vi "Confirm Device UI.vi"(11 "Device":refnum<class "Device.lvclass">) -> (3 "Confirmed":bool)   [LabVIEW 2020, in "PicoG-App.lvlib" / "picoG.lvclass"]
uses:
  picoG.lvclass
  Device/Device.lvclass
panel:
  out "Picture":picture
  in  "Cancel Button":bool
  in  "OK Button":bool
  out "Version":string
  out "Name":string
  out "Id / Serial":string
  out "Board":string
  out "Platform":string
  # "Confirm device selection to continue adding the device to the registry.\n\nIf desired, the alias can be changed once the device is added."
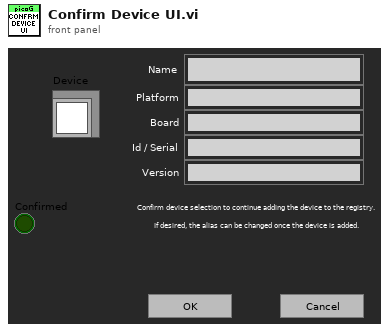
[diagram p1: front panel]
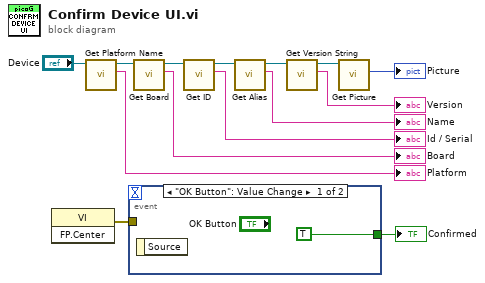
[diagram p0: block diagram]
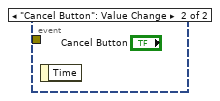
[diagram p2: hidden frame]
diagram:
  n1 = invoke class="VI" method="FP.Center"() -> (error out=w3:errorcluster)  [unwired: 3 in, 2 out]
  n2 = call "Get Platform Name.vi"("Device in"="Device") -> ("Platform"=→"Platform":string, "Device out"=w13:refnum<class "Device.lvclass">)  [unwired: 8 in, 1 out]
  n3 = event shown="[0] \"OK Button\": Value Change" {
    selector: _ -> [_ _]
    dyn-events: _ -> [_ _]
    timeout: _ -> [_ _]
    tunnel: [TRUE _] -> w4
    tunnel: w3 -> [_ _]
    event "OK Button": Value Change {
      n4 = event-data() -> ()  [unwired: 1 in, 1 out]
    }
    event "Cancel Button": Value Change {
      n5 = event-data() -> ()  [unwired: 1 in, 1 out]
    }
  }
  "Confirmed" <- w4
  n6 = call "Get Board.vi"("Device in"=w13) -> ("Board"=→"Board":string, "Device out"=w12:refnum<class "Device.lvclass">)  [unwired: 8 in, 1 out]
  n7 = call "Get ID.vi"("Device in"=w12) -> ("Id"=→"Id / Serial":string, "Device out"=w11:refnum<class "Device.lvclass">)  [unwired: 8 in, 1 out]
  n8 = call "Get Alias.vi"("Device in"=w11) -> ("Alias"=→"Name":string, "Device out"=w10:refnum<class "Device.lvclass">)  [unwired: 8 in, 1 out]
  n9 = call "Get Version String.vi"("Device in"=w10) -> ("Version"=→"Version":string, "Device out"=w2:refnum<class "Device.lvclass">)  [unwired: 8 in, 1 out]
  n10 = call "Get Picture.vi"("Device in"=w2) -> ("Picture"=→"Picture":picture)  [unwired: 8 in, 2 out]
